vi "Init Data.vi"(8 "error in (no error)":errorcluster, 10 "Array of TriggerAction Elements":T1[](array[typedef]), 11 "TriggerAction in":refnum<class "TriggerAction Q.lvclass">) -> (0 "error out":errorcluster, 3 "TriggerAction out":refnum<class "TriggerAction Q.lvclass">)   [LabVIEW 2016, in "TriggerAction Q.lvclass"]
uses:
  <userlib>/Common Components/TriggerAction Q/TriggerAction Q/TriggerAction Q.lvclass
  <userlib>/Common Components/TriggerAction Q/TriggerAction Q/Element Data.ctl
  <userlib>/Common Components/TriggerAction Q/TriggerAction Q/TriggerAction Q.lvclass/TriggerAction Q.ctl
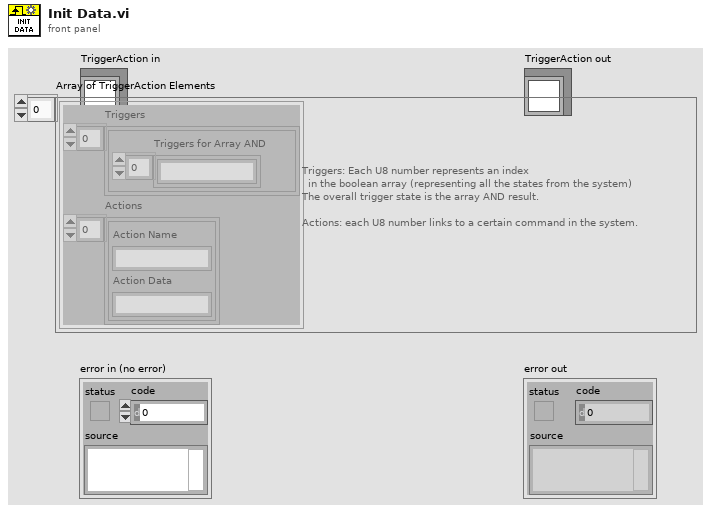
[diagram p1: front panel]
types:
  T1 = typedef "TriggerAction Q.lvclass/Element Data.ctl" = cluster{"Triggers":cluster{"Triggers for Array AND":string[]}[], "Actions":cluster{"Action Name":string, "Action Data":string}[]}
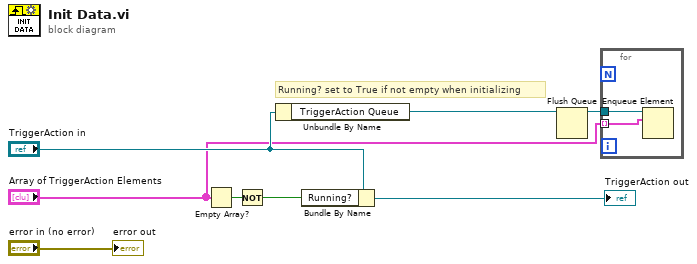
[diagram p0: block diagram]
diagram:
  # "Running? set to True if not empty when initializing"
  n1 = Empty Array?(array="Array of TriggerAction Elements") -> (empty?=w2:bool)
  n2 = Not(x=w2) -> (.not. x?=w1:bool)
  n3 = Unbundle By Name("TriggerAction in") -> ("TriggerAction Queue"=w6:refnum<queue>)
  n4 = Bundle By Name(cluster="TriggerAction in", "Running?"=w1) -> (→"TriggerAction out":refnum<class "TriggerAction Q.lvclass">)
  n5 = Flush Queue(queue=w6) -> (queue out=w5:refnum<queue>)  [unwired: 1 in, 2 out]
  n6 = for {
    tunnel: w5 -> [w10]
    tunnel: "Array of TriggerAction Elements" -> [w9] mode=indexing
    n7 = Enqueue Element(queue=w10, element=w9) -> ()  [unwired: 2 in, 3 out]
  }
  "error out" <- "error in (no error)"
